vi "Get Active VI of Runtime App Ref.vi"(8 "error in (no error)":errorcluster, 11 "App Ref":refnum<vi>) -> (0 "error out":errorcluster, 3 "Active VI Ref":refnum<vi>)   [LabVIEW 2020, in "MacroAssert.lvlib"]
doc: "Gets the active (or frontmost) VI within <B>App Ref</B> in the situation where App.Kind is Run Time Engine."
uses:
  MacroAssert.lvlib
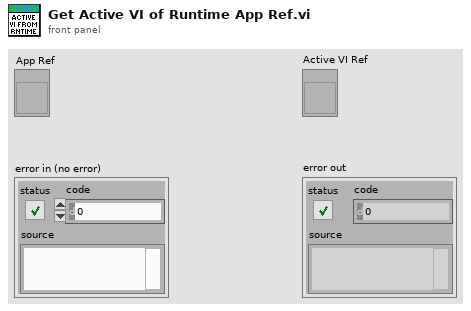
[diagram p1: front panel]
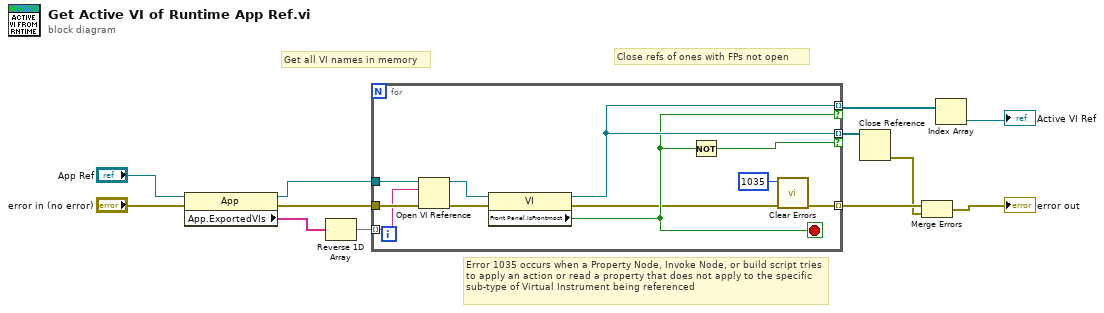
[diagram p0: block diagram]
diagram:
  # "Error 1035 occurs when a Property Node, Invoke Node, or build script tries to apply an action or read a property that does not apply to the specific sub-type of Virtual Instrument being referenced"
  # "Get all VI names in memory"
  # "Close refs of ones with FPs not open"
  n1 = property class="App"(reference="App Ref", error in="error in (no error)") -> (reference out=w5:refnum<vi>, error out=w8:errorcluster, "App.ExportedVIs"=w7:string[])
  n2 = Reverse 1D Array(array=w7) -> (reversed array=w1:string[])
  n3 = for {
    tunnel: [w18] -> w12 mode=indexing if=w17
    tunnel: [w18] -> w4 mode=indexing if=w16
    tunnel: w8 -> [w23]
    tunnel: [w13] -> w11 mode=indexing
    tunnel: w5 -> [w22]
    tunnel: w1 -> [w21] mode=indexing
    stop <- w16 stop-if-true
    n4 = Open VI Reference(application reference (local)=w22, vi path=w21, error in (no error)=w23) -> (vi reference=w19:refnum<vi>, error out=w20:errorcluster)  [unwired: 3 in]
    n5 = property class="VI"(reference=w19, error in=w20) -> (reference out=w18:refnum<vi>, error out=w14:errorcluster, "Front Panel.IsFrontmost"=w16:bool)
    n6 = Not(x=w16) -> (.not. x?=w17:bool)
    n7 = call <vilib>:"Clear Errors.vi"("error in (no error)"=w14, "specific error code to clear (0: all)"=1035) -> ("error out"=w13:errorcluster)  [unwired: 4 in, 1 out]
  }
  n8 = Close Reference(reference=w12) -> (error out=w6:errorcluster)  [unwired: 1 in]
  n9 = Merge Errors(w11, w6) -> (→"error out":errorcluster)
  n10 = Index Array(array=w4) -> (element=→"Active VI Ref":refnum<vi>)  [unwired: 1 in]
